vi "ABB bearing rdgs.vi"(6 "Run Time":dbl, 7 "Site ambient":dbl=40.0, 8 "Readings in":dbl[][](array[numeric]), 9 "Aditional temps":dbl[](array[numeric]), 10 "temperatures":dbl[](array[numeric]), 11 "Primary coolant":u16(ring) items=["Oil", "Water", "Natural"]) -> (0 "Readings out":dbl[][](array[numeric]), 1 "NDE rise":dbl, 2 "Temperature trend":cluster{dbl[], dbl[]}[](array[cluster]), 4 "DE rise":dbl, 5 "rise rate":dbl)   [LabVIEW 2017]
panel:
  out "Final bearing temp rise (degree K)":dbl
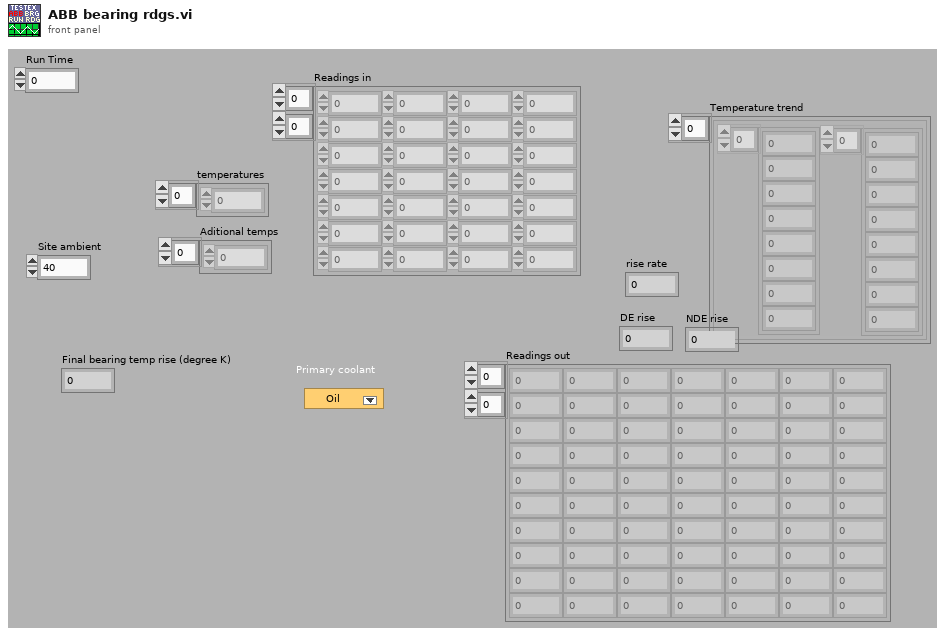
[diagram p1: front panel]
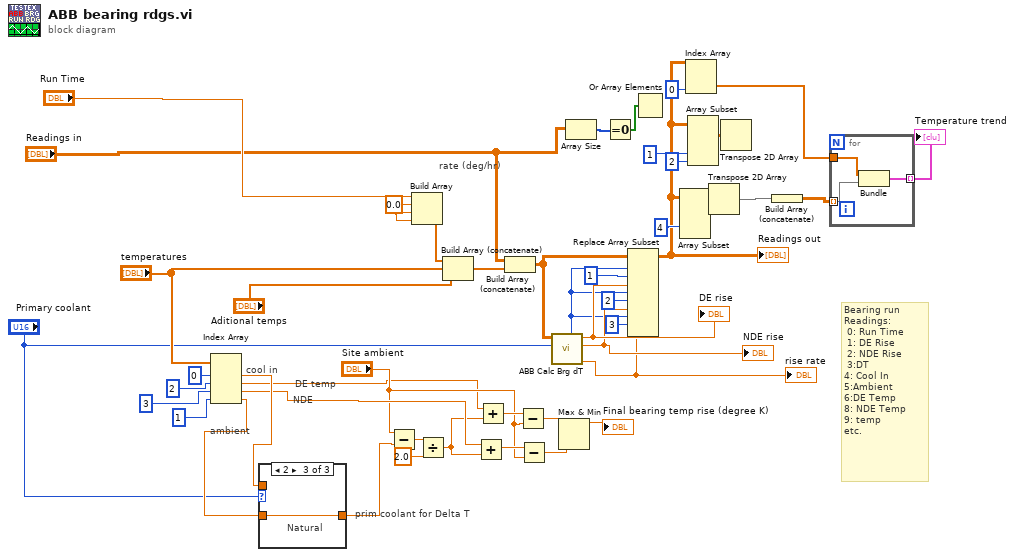
[diagram p0: block diagram]
diagram:
  w7 = 0.0 ("element")
  # "Bearing run Readings:\n 0: Run Time\n 1: DE Rise\n 2: NDE Rise\n 3:DT\n4: Cool In\n5:Ambient\n6:DE Temp\n8: NDE Temp\n9: temp\netc."
  # "prim coolant for Delta T"
  # "ambient"
  # "NDE"
  # "rate (deg/hr)"
  # "cool in"
  # "DE temp"
  n1 = Index Array(array="temperatures", index #1=0 ("index"), index #2=2 ("index"), index #3=3 ("index"), index #4=1 ("index")) -> (element #1=w34:dbl, element #2=w26:dbl, element #3=w31:dbl, element #4=w35:dbl)
  n2 = case shown="2" "Primary coolant" {
    tunnel: w35 -> [_ _ w50]
    tunnel: [w48 w49 w50] -> w22
    tunnel: w34 -> [w48 w49 _]
    frame 0, Default {
      # "Oil"
    }
    frame 1 {
      # "Water"
    }
    frame 2 {
      # "Natural"
    }
  }
  n3 = Subtract(x="Site ambient", y=w22) -> (x-y=w33:dbl)
  n4 = Build Array("Run Time", w7, w7, w7) -> (w39:dbl[])
  n5 = Divide(x=w33, y=2.0) -> (x/y=w30:dbl)
  n6 = Build Array (concatenate)(w39, "temperatures", "Aditional temps") -> (w43:dbl[])
  n7 = Add(x=w31, y=w30) -> (x+y=w28:dbl)
  n8 = Add(x=w26, y=w30) -> (x+y=w29:dbl)
  n9 = Build Array (concatenate)("Readings in", w43) -> (w17:dbl[][])
  n10 = Subtract(x=w29, y="Site ambient") -> (x-y=w25:dbl)
  n11 = Subtract(x=w28, y="Site ambient") -> (x-y=w24:dbl)
  n12 = call "ABB Calc Brg dT.vi"("Primary coolant"="Primary coolant", "Readings in"=w17) -> ("dT (deg/hr)"=w8:dbl, "NDE rise"=w11:dbl, "DE rise"=w12:dbl, "lastindex"=w10:i32)  [unwired: 5 in, 1 out]
  "rise rate" <- w8
  "DE rise" <- w12
  "NDE rise" <- w11
  n13 = Max & Min(x=w25, y=w24) -> (max(x,y)=→"Final bearing temp rise (degree K)":dbl)  [unwired: 1 out]
  n14 = Array Size(array="Readings in") -> (size(s)=w20:i32[])
  n15 = Equal To 0?(x=w20) -> (x = 0?=w19:bool[])
  n16 = Replace Array Subset(array=w17, new element #1=w12, index (row) #1=w10, index (col) #1=1 ("disabled index (col)"), new element #2=w11, index (row) #2=w10, index (col) #2=2 ("disabled index (col)"), new element #3=w8, index (row) #3=w10, index (col) #3=3 ("disabled index (col)")) -> (w15:dbl[][])
  "Readings out" <- w15
  n17 = Or Array Elements(Boolean array=w19) -> ()  [unwired: 1 out]
  n18 = Array Subset(array=w15, index (col)=4 ("index")) -> (w4:dbl[][])  [unwired: 3 in]
  n19 = Index Array(array=w15, index (col)=0 ("disabled index (col)")) -> (element=w45:dbl[])  [unwired: 1 in]
  n20 = Array Subset(array=w15, index (col)=1 ("disabled index (col)"), length (col)=2 ("length")) -> (w37:dbl[][])  [unwired: 2 in]
  n21 = Transpose 2D Array(2D array=w4) -> (transposed array=w3:dbl[][])
  n22 = Transpose 2D Array(2D array=w37) -> ()  [unwired: 1 out]
  n23 = Build Array (concatenate)(w3) -> (w2:dbl[][])
  n24 = for {
    tunnel: w45 -> [w53]
    tunnel: w2 -> [w52] mode=indexing
    tunnel: [w51] -> w47 mode=indexing
    n25 = Bundle(w53, w52) -> (w51:cluster{dbl[], dbl[]})  [unwired: 1 in]
  }
  "Temperature trend" <- w47
